vi "Create TimerDRV.vi"(8 "error in (no error)":errorcluster, 10 "Trigger ID":u8=100) -> (0 "error out":errorcluster, 3 "TimerDRV out":refnum<class "TimerDRV.lvclass">)   [LabVIEW 2019, in "TimingDRV Engine.lvlib" / "TimerDRV.lvclass"]
uses:
  TimerDRV.lvclass
  TypeDefs/Command Package.ctl
  TypeDefs/Command.ctl
  TimerDRV.lvclass/TimerDRV.ctl
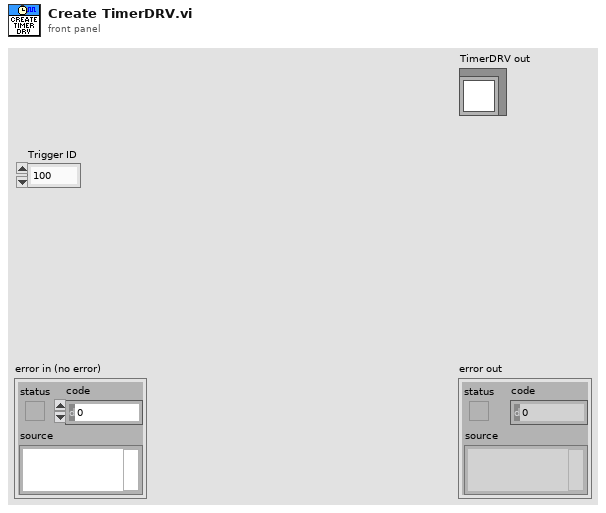
[diagram p1: front panel]
types:
  T1 = typedef "TimingDRV Engine.lvlib/TimerDRV.lvclass/Command Package.ctl" = cluster{"Command":T2, "Command Data":variant}
  T2 = typedef "TimingDRV Engine.lvlib/TimerDRV.lvclass/Command.ctl" = enum16{"Shutdown", "Update Execution Frequency", "Initialize"}
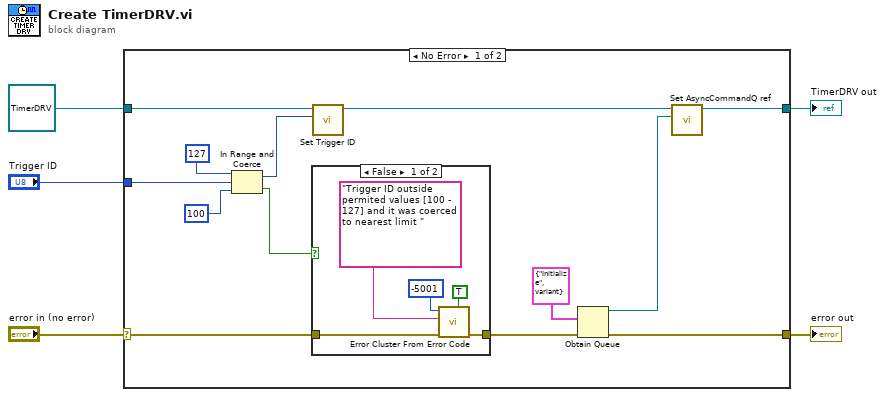
[diagram p0: block diagram]
diagram:
  n1 = case shown="No Error" "error in (no error)" {
    selector: "error in (no error)" -> [w10 w26]
    tunnel: [w7 w26] -> w4
    tunnel: [w17 w25] -> w2
    tunnel: refnum<class "TimerDRV.lvclass"> refnum ("TimerDRV in") -> [w16 w25]
    tunnel: "Trigger ID" -> [w14 _]
    frame No Error {
      n2 = In Range and Coerce(upper limit=u8 127, x=w14, lower limit=u8 100) -> (coerced(x)=w11:u8, In Range?=w8:bool)
      n3 = case shown="False" w8 {
        tunnel: w10 -> [w23 w24]
        tunnel: [w22 w24] -> w9
        frame False {
          n4 = call <vilib>:"Error Cluster From Error Code.vi"("is warning? (False)"=TRUE, "error in (no error)"=w23, "error message (\"\")"="Trigger ID outside permited values [100 - 127] and it was coerced to nearest limit " ("error message (\"\")"), "error code (0)"=-5001) -> ("error out"=w22:errorcluster)  [unwired: 5 in]
        }
        frame True {
        }
      }
      n5 = call "Set Trigger ID.vi"("Trigger ID"=w11, "TimerDRV in"=w16) -> ("TimerDRV out"=w15:refnum<class "TimerDRV.lvclass">)  [unwired: 9 in]
      n6 = Obtain Queue(element data type=T1 {"Command"=enum."Initialize", "Command Data"=variant}, error in (no error)=w9) -> (queue out=w6:refnum<queue>, error out=w7:errorcluster)  [unwired: 3 in, 1 out]
      n7 = call "Set AsyncCommandQ ref.vi"("AsyncCommandQ"=w6, "TimerDRV in"=w15) -> ("TimerDRV out"=w17:refnum<class "TimerDRV.lvclass">)  [unwired: 9 in]
    }
    frame Error {
    }
  }
  "error out" <- w4
  "TimerDRV out" <- w2
